vi "get Device Number.vi"(11 "instanceNumber":i32) -> (3 "function return":u32)   [LabVIEW 2022 SP3, in "SADI_FW3.lvlib"]
doc: "SADI_API unsigned int getDeviceNumber(int instanceNumber);\nSADI_API unsigned int getDeviceNumber(int instanceNumber);"
uses:
  SADI_FW3.lvlib
  SADI_FW3.dll
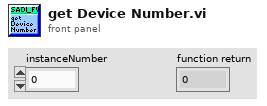
[diagram p1: front panel]
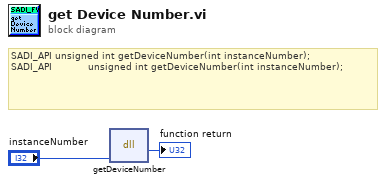
[diagram p0: block diagram]
diagram:
  # "SADI_API unsigned int getDeviceNumber(int instanceNumber);\nSADI_API            unsigned int getDeviceNumber(int instanceNumber);"
  n1 = dll-call lib="C:/Users/scer/OneDrive - University of Florida/eml4314c/eml4314Sp24/Resources/release_1_11_24/EML4314c_Sp24_framework_0/LVLib/SADI_FW3.*" fn="getDeviceNumber"("instanceNumber"="instanceNumber") -> (→"function return":u32)  [unwired: 4 in, 2 out]
